vi "多态-动作检查.vi"   [LabVIEW 2017, in "调试与报错.lvlib"]
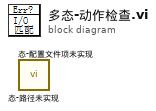
[diagram p0: block diagram]
diagram:
  n1 = call "态-路径未实现.vi"() -> ()  [unwired: 9 in, 3 out]
  n2 = call "态-配置文件项未实现.vi"() -> ()  [unwired: 9 in, 3 out]
